vi "ws Spartan Version.vi"() -> (1 "Version":T1={"Version"="5.2", "Build Number"=202, "Build Date/Time"=3349904508.0749164} {"Build Date/Time" format="%<%X\n%x>T"})   [LabVIEW 2011]
uses:
  SI.LIB/OGAB Version.ctl
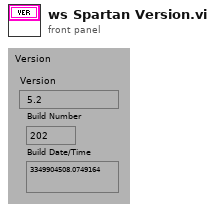
[diagram p1: front panel]
types:
  T1 = typedef "OGAB Version.ctl" = cluster{"Version":string, "Build Number":u32, "Build Date/Time":dbl}
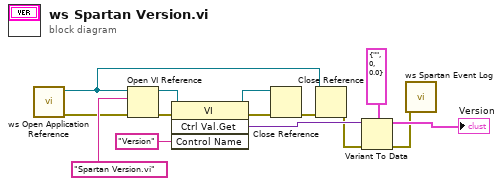
[diagram p0: block diagram]
diagram:
  n1 = call "ws Open Application Reference.vi"() -> ("error out"=w4:errorcluster, "application reference"=w3:refnum<vi>)  [unwired: 10 in]
  n2 = Open VI Reference(application reference (local)=w3, vi path="Spartan Version.vi", error in (no error)=w4) -> (vi reference=w6:refnum<vi>, error out=w7:errorcluster)  [unwired: 3 in]
  n3 = invoke class="VI" method="Ctrl Val.Get"(reference=w6, error in=w7, "Control Name"="Version") -> (reference out=w10:refnum<vi>, error out=w11:errorcluster, "Get Control Value Variant"=w12:variant)  [unwired: 1 in, 1 out]
  n4 = Close Reference(reference=w10, error in (no error)=w11) -> (error out=w5:errorcluster)
  n5 = Close Reference(reference=w3, error in (no error)=w5) -> (error out=w2:errorcluster)
  n6 = Variant To Data(error in=w2, type=T1 {"Version"="", "Build Number"=0, "Build Date/Time"=0.0} ("CONFIG"), Variant=w12) -> (data=→"Version":T1, error out=w1:errorcluster)
  n7 = call "ws Spartan Event Log.vi"("error in (no error)"=w1) -> ()  [unwired: 7 in, 1 out]
